vi "WriteTxtDataAnaFile_DP_ver1.0.vi"(2 "2D Data Array In":dbl[][](array[numeric]), 4 "error in":errorcluster, 7 "file path":path) -> (0 "error out":errorcluster)   [LabVIEW 2012]
doc: "Input 2D data array and Data Save Info. Then, save all the data and info. in Igor format. If \"Title Name Array\" is empty, the title name in igor file would be the title name column from \"Instrs configs 2D arrary\""
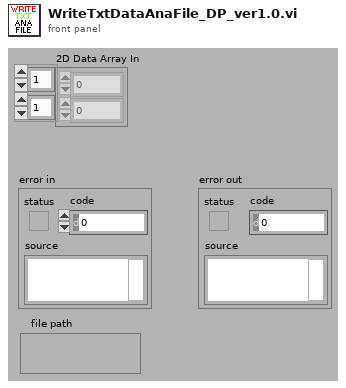
[diagram p1: front panel]
types:
  T1 = enum16{"open", "open or create", "create or replace", "create", "open (read only)"}
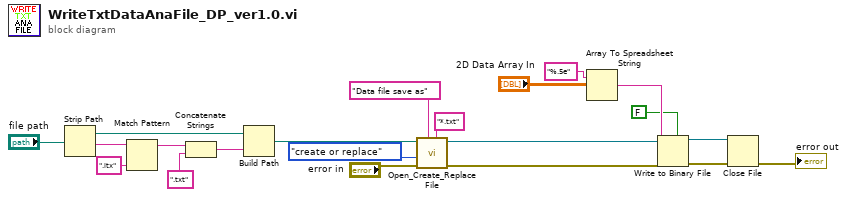
[diagram p0: block diagram]
diagram:
  n1 = Strip Path(path="file path") -> (stripped path=w5:path, name=w12:string)
  n2 = Match Pattern(string=w12, regular expression=".itx") -> (before substring=w6:string)  [unwired: 1 in, 3 out]
  n3 = Concatenate Strings(w6, ".txt" ("format string")) -> (w10:string)
  n4 = Build Path(base path=w5, name or relative path=w10) -> (appended path=w9:path)
  n5 = call <vilib>:"Open_Create_Replace File.vi"("pattern"="*.txt", "prompt"="Data file save as", "error in (no error)"="error in", "function (open:0)"=T1."create or replace", "file path"=w9) -> ("error out"=w7:errorcluster, "refnum"=w8:refnum<file>)  [unwired: 2 in, 3 out]
  n6 = Array To Spreadsheet String(array="2D Data Array In", 3:"%.5e" ("format string")) -> (spreadsheet string=w20:string)  [unwired: 1 out]
  n7 = Write to Binary File(file (use dialog)=w8, data=w20, error in=w7, 5:FALSE ("prepend array or string size? (T)")) -> (refnum out=w2:refnum<file>, error out=w3:errorcluster)  [unwired: 3 out]
  n8 = Close File(refnum=w2, error in=w3) -> (error out=→"error out":errorcluster)  [unwired: 1 out]
